vi "SubVI_CreateBottom.vi"(5 "BP_Point(0,0)":cluster{"Width":i32, "Height":i32}={"Width"=0, "Height"=36}, 6 "Ref位移":i32=100, 7 "FP_Point(0,0)":cluster{"Width":i32, "Height":i32}, 8 "error in (no error)":errorcluster, 9 "Value":string[](array[string]), 11 "VI in":refnum<vi>) -> (0 "error out":errorcluster, 2 "Array":refnum<vi>[](array[refnum]), 3 "VI out":refnum<vi>)   [LabVIEW 2015]
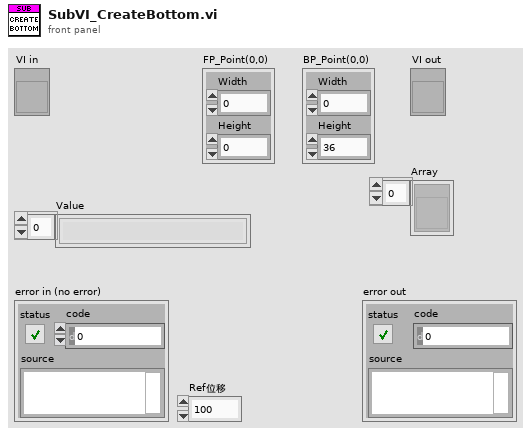
[diagram p1: front panel]
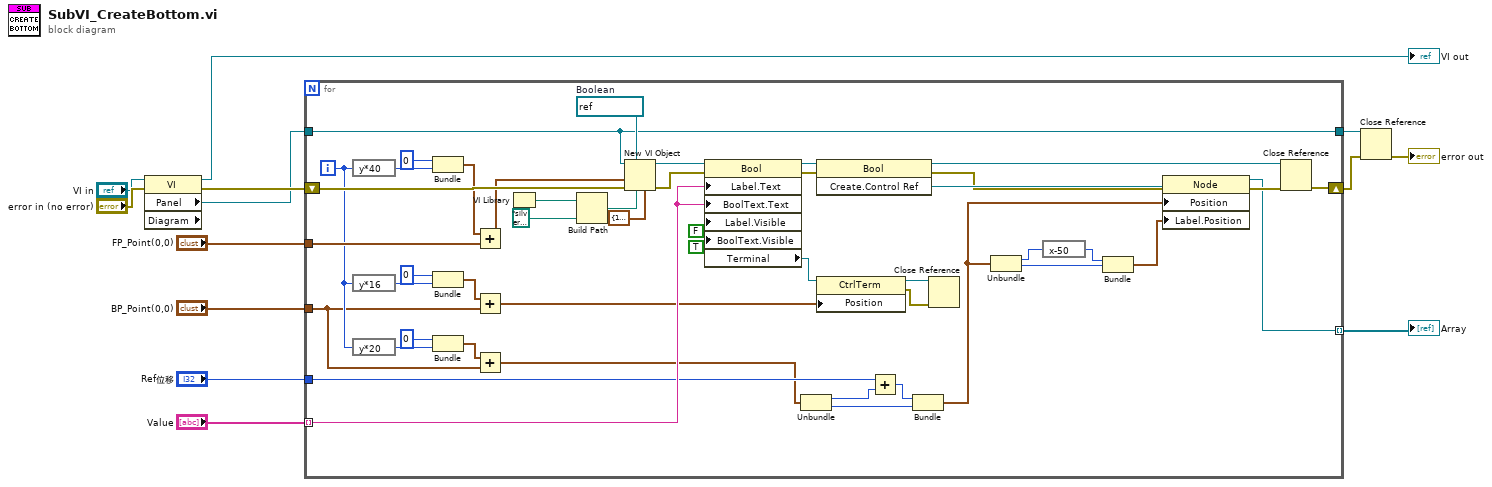
[diagram p0: block diagram]
diagram:
  n1 = property class="VI" props=["Panel", "Diagram"](reference="VI in", error in="error in (no error)") -> (reference out=→"VI out":refnum<vi>, error out=w5:errorcluster, "Panel"=w4:refnum<vi>)  [unwired: 1 out]
  n2 = for {
    tunnel: w4 -> [w49]
    tunnel: "Value" -> [w54] mode=indexing
    shift-right: [w42] -> w2
    shift-left: w5 -> [w44]
    tunnel: [w49] -> w3
    tunnel: [w37] -> w1 mode=indexing
    tunnel: "FP_Point(0,0)" -> [w35]
    tunnel: "BP_Point(0,0)" -> [w16]
    tunnel: "Ref位移" -> [w28]
    i -> [w18]
    w60 = refnum<vi> refnum  # Boolean
    n3 = expression code="y*40"(w18) -> (w51:i32)
    n4 = expression code="y*16"(w18) -> (w25:i32)
    n5 = expression code="y*20"(w18) -> (w20:i32)
    n6 = Bundle(0, w51) -> (w34:cluster{i32, i32})  [unwired: 1 in]
    n7 = Bundle(0, w25) -> (w26:cluster{i32, i32})  [unwired: 1 in]
    n8 = Bundle(0, w20) -> (w19:cluster{i32, i32})  [unwired: 1 in]
    n9 = Add(x=w34, y=w35) -> (x+y=w33:cluster{i32, i32})
    n10 = Add(x=w26, y=w16) -> (x+y=w32:cluster{i32, i32})
    n11 = Add(x=w19, y=w16) -> (x+y=w15:cluster{i32, i32})
    n12 = VI Library() -> (path=w57:path)
    n13 = Build Path(base path=w57, name or relative path=path "silver_ctls/Boolean/Blank Button NI_Silver.ctl" ("path")) -> (appended path=w56:path)
    n14 = New VI Object(vi object class=w60, owner refnum=w49, position/next to=w33, 4:cluster{"Width":u32, "Height":u32} {"Width"=100, "Height"=36}, 6:w56, 8:w44) -> (object refnum=w59:refnum<vi>, 0:w58:errorcluster)  [unwired: 2 in]
    n15 = property class="Bool"(reference=w59, error in=w58, "Label.Text"=w54, "BoolText.Text"=w54, "Label.Visible"=FALSE, "BoolText.Visible"=TRUE ("Label.Visible")) -> (reference out=w48:refnum<vi>, error out=w45:errorcluster, "Terminal"=w41:refnum<vi>)
    n16 = Unbundle(w15) -> (w30:i32, w36:i32)
    n17 = invoke class="Bool" method="Create.Control Ref"(reference=w48, error in=w45) -> (reference out=w47:refnum<vi>, error out=w43:errorcluster, "Create Control Ref"=w46:refnum<vi>)  [unwired: 1 in]
    n18 = property class="CtrlTerm"(reference=w41, "Position"=w32) -> (reference out=w40:refnum<vi>, error out=w39:errorcluster)  [unwired: 1 in]
    n19 = Add(x=w28, y=w30) -> (x+y=w29:i32)
    n20 = Bundle(w29, w36) -> (w24:cluster{i32, i32})  [unwired: 1 in]
    n21 = Close Reference(reference=w40, error in (no error)=w39) -> ()  [unwired: 1 out]
    n22 = Unbundle(w24) -> (w22:i32, w14:i32)
    n23 = expression code="x-50"(w22) -> (w23:i32)
    n24 = Bundle(w23, w14) -> (w21:cluster{i32, i32})  [unwired: 1 in]
    n25 = property class="Node"(reference=w46, error in=w43, "Position"=w24, "Label.Position"=w21) -> (reference out=w37:refnum<vi>, error out=w38:errorcluster)
    n26 = Close Reference(reference=w47, error in (no error)=w38) -> (error out=w42:errorcluster)
  }
  "Array" <- w1
  n27 = Close Reference(reference=w3, error in (no error)=w2) -> (error out=→"error out":errorcluster)
